vi "Add Library To Project.vi"(8 "error in":errorcluster, 10 "library path":path, 11 "Config":T1) -> (0 "error out":errorcluster, 3 "project ref out":refnum<vi>)   [LabVIEW 2021, in "G-Plugin Editor.lvlib"]
uses:
  G-Plugin Editor.lvlib
  controls/Data Holder.ctl
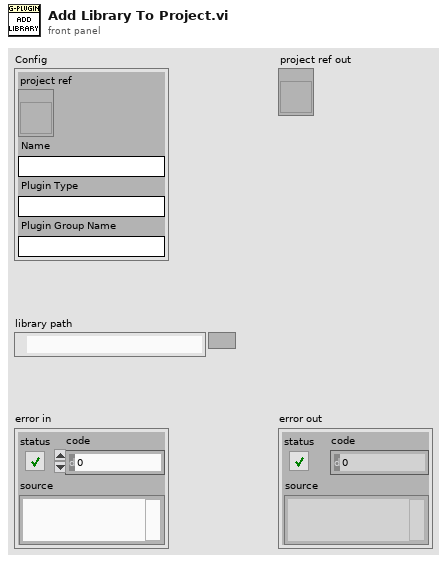
[diagram p1: front panel]
types:
  T1 = typedef "G-Plugin Editor.lvlib/Data Holder.ctl" = cluster{"project ref":refnum<vi>, "Name":string, "Plugin Type":string, "Plugin Group Name":string}
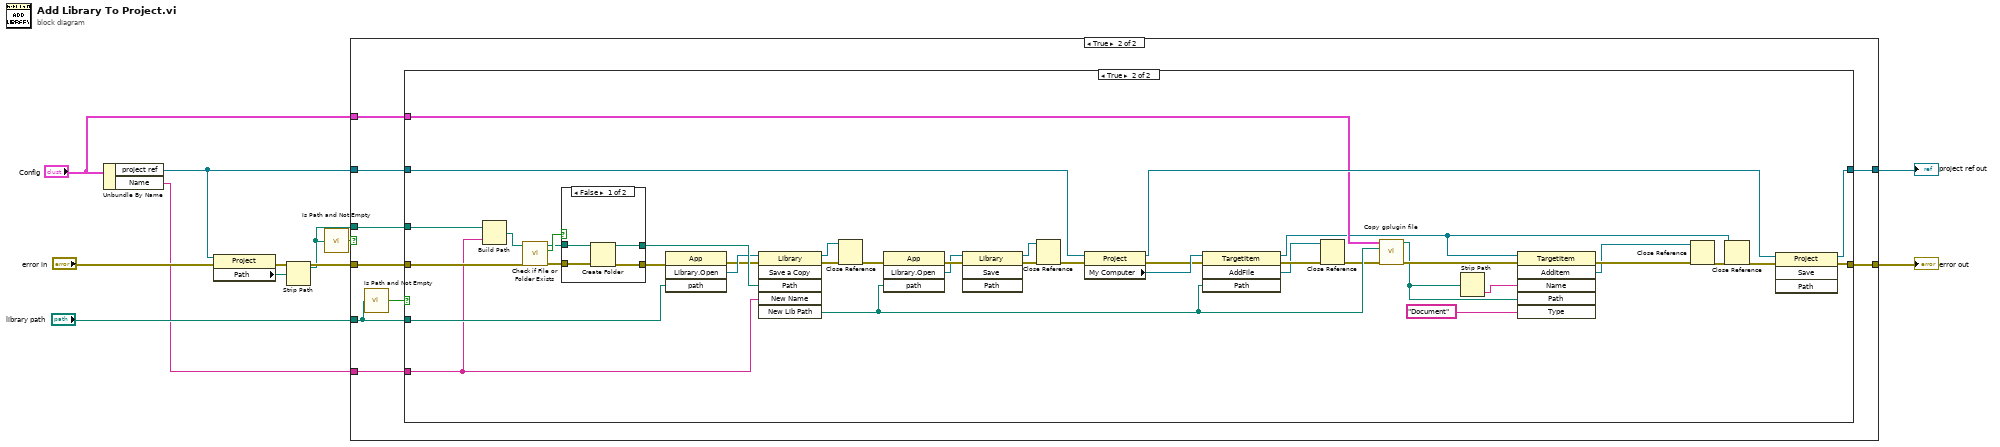
[diagram p0: block diagram]
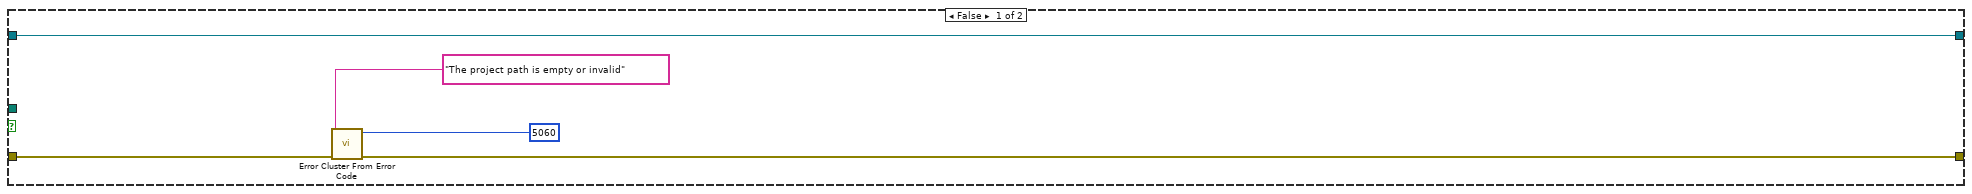
[diagram p2: hidden frame]
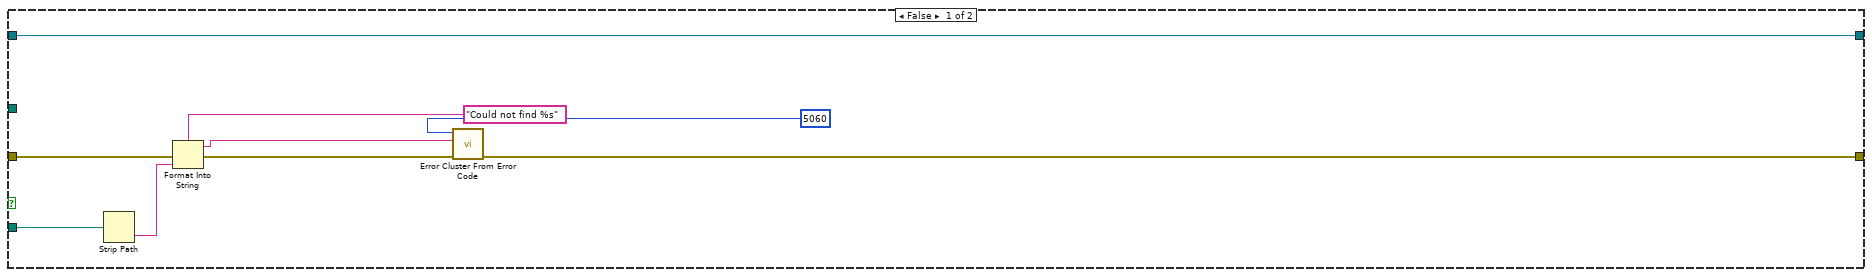
[diagram p3: hidden frame]
diagram:
  n1 = Unbundle By Name("Config") -> ("project ref"=w3:refnum<vi>, "Name"=w2:string)
  n2 = property class="Project"(reference=w3, error in="error in") -> (error out=w8:errorcluster, "Path"=w7:path)  [unwired: 1 out]
  n3 = Strip Path(path=w7) -> (stripped path=w6:path)  [unwired: 1 out]
  n4 = call <vilib>:"Is Path and Not Empty.vi"("path"=w6) -> ("Is Path and Not Empty?"=w11:bool)  [unwired: 4 in]
  n5 = case shown="True" w11 {
    tunnel: w8 -> [w16 w25]
    tunnel: [w15 w24] -> w10
    tunnel: "library path" -> [_ w22]
    tunnel: w2 -> [_ w21]
    tunnel: w6 -> [_ w20]
    tunnel: w3 -> [w12 w19]
    tunnel: [w12 w18] -> w4
    tunnel: "Config" -> [_ w17]
    frame False {
      n6 = call <vilib>:"Error Cluster From Error Code.vi"("error in (no error)"=w16, "error message (\"\")"="The project path is empty or invalid" ("error message (\"\")"), "error code (0)"=5060) -> ("error out"=w15:errorcluster)  [unwired: 6 in]
    }
    frame True {
      n7 = call <vilib>:"Is Path and Not Empty.vi"("path"=w22) -> ("Is Path and Not Empty?"=w23:bool)  [unwired: 4 in]
      n8 = case shown="True" w23 {
        tunnel: w25 -> [w33 w74]
        tunnel: [w32 w72] -> w24
        tunnel: w22 -> [w29 w73]
        tunnel: w21 -> [_ w63]
        tunnel: w20 -> [_ w71]
        tunnel: w19 -> [w26 w70]
        tunnel: [w26 w48] -> w18
        tunnel: w17 -> [_ w46]
        frame False {
          n9 = Strip Path(path=w29) -> (name=w30:string)  [unwired: 1 out]
          n10 = Format Into String(format string="Could not find %s", error in=w33, w30) -> (resulting string=w27:string, error out=w31:errorcluster)  [unwired: 1 in]
          n11 = call <vilib>:"Error Cluster From Error Code.vi"("error in (no error)"=w31, "error message (\"\")"=w27, "error code (0)"=5060) -> ("error out"=w32:errorcluster)  [unwired: 6 in]
        }
        frame True {
          n12 = Build Path(base path=w71, name or relative path=w63) -> (appended path=w69:path)
          n13 = call <vilib>:"Check if File or Folder Exists.vi"("error in (no error)"=w74, "path"=w69) -> ("error out"=w66:errorcluster, "file or folder exists?"=w68:bool, "dup path"=w67:path)  [unwired: 7 in]
          n14 = case shown="False" w68 {
            tunnel: w67 -> [w77 w80]
            tunnel: w66 -> [w78 w79]
            tunnel: [w76 w79] -> w65
            tunnel: [w75 w80] -> w64
            frame False {
              n15 = Create Folder(path (use dialog)=w77, error in=w78) -> (created path=w75:path, error out=w76:errorcluster)  [unwired: 1 in, 1 out]
            }
            frame True {
            }
          }
          n16 = invoke class="App" method="Library.Open"(error in=w65, "path"=w73) -> (error out=w53:errorcluster, "Open Library"=w62:refnum<vi>)  [unwired: 2 in, 2 out]
          n17 = invoke class="Library" method="Save a Copy"(reference=w62, error in=w53, "Path"=w64, "New Name"=w63) -> (reference out=w58:refnum<vi>, error out=w60:errorcluster, "New Lib Path"=w47:path)  [unwired: 2 in, 3 out]
          n18 = Close Reference(reference=w58, error in (no error)=w60) -> (error out=w59:errorcluster)
          n19 = invoke class="App" method="Library.Open"(error in=w59, "path"=w47) -> (error out=w50:errorcluster, "Open Library"=w49:refnum<vi>)  [unwired: 2 in, 2 out]
          n20 = invoke class="Library" method="Save"(reference=w49, error in=w50) -> (reference out=w56:refnum<vi>, error out=w57:errorcluster)  [unwired: 2 in, 2 out]
          n21 = Close Reference(reference=w56, error in (no error)=w57) -> (error out=w55:errorcluster)
          n22 = property class="Project"(reference=w70, error in=w55) -> (reference out=w54:refnum<vi>, error out=w45:errorcluster, "My Computer"=w61:refnum<vi>)
          n23 = invoke class="TargetItem" method="AddFile"(reference=w61, error in=w45, "Path"=w47) -> (reference out=w36:refnum<vi>, error out=w43:errorcluster, "AddFile"=w37:refnum<vi>)  [unwired: 1 in, 1 out]
          n24 = Close Reference(reference=w37, error in (no error)=w43) -> (error out=w42:errorcluster)
          n25 = call "Copy gplugin file.vi"("Config"=w46, "Plugin Path"=w47, "error in (no error)"=w42) -> ("G PLugin File Path"=w39:path, "error out"=w44:errorcluster)  [unwired: 11 in]
          n26 = Strip Path(path=w39) -> (name=w38:string)  [unwired: 1 out]
          n27 = invoke class="TargetItem" method="AddItem"(reference=w36, error in=w44, "Name"=w38, "Path"=w39, "Type"="Document") -> (error out=w40:errorcluster, "AddItem"=w35:refnum<vi>)  [unwired: 1 in, 4 out]
          n28 = Close Reference(reference=w35, error in (no error)=w40) -> (error out=w52:errorcluster)
          n29 = Close Reference(reference=w36, error in (no error)=w52) -> (error out=w51:errorcluster)
          n30 = invoke class="Project" method="Save"(reference=w54, error in=w51) -> (reference out=w48:refnum<vi>, error out=w72:errorcluster)  [unwired: 2 in, 2 out]
        }
      }
    }
  }
  "error out" <- w10
  "project ref out" <- w4
